vi "Get Last10 Data.vi"(8 "error in (no error)":errorcluster, 11 "Ref In":T1 {"TS Parameter"."FCA" format="%01d"; "TS Parameter"."Target" min=1 max=100000; "TS Parameter"."PokaYoke" min=0 max=1}) -> (0 "error out":errorcluster, 3 "Ref Out":T1 {"TS Parameter"."FCA" format="%01d"; "TS Parameter"."Target" min=1 max=100000; "TS Parameter"."PokaYoke" min=0 max=1}, 4 "BCODE SLNO":i32, 6 "Table Control":string[][](array[string]))   [LabVIEW 2020]
uses:
  Controls/TD SQL.ctl
  <vilib>/addons/database/Connection.llb/Conn ObjectReference.ctl
  Controls/WIP_State.ctl
  Controls/TS_Parameter.ctl
  <vilib>/addons/database/NI_Database_API.lvlib
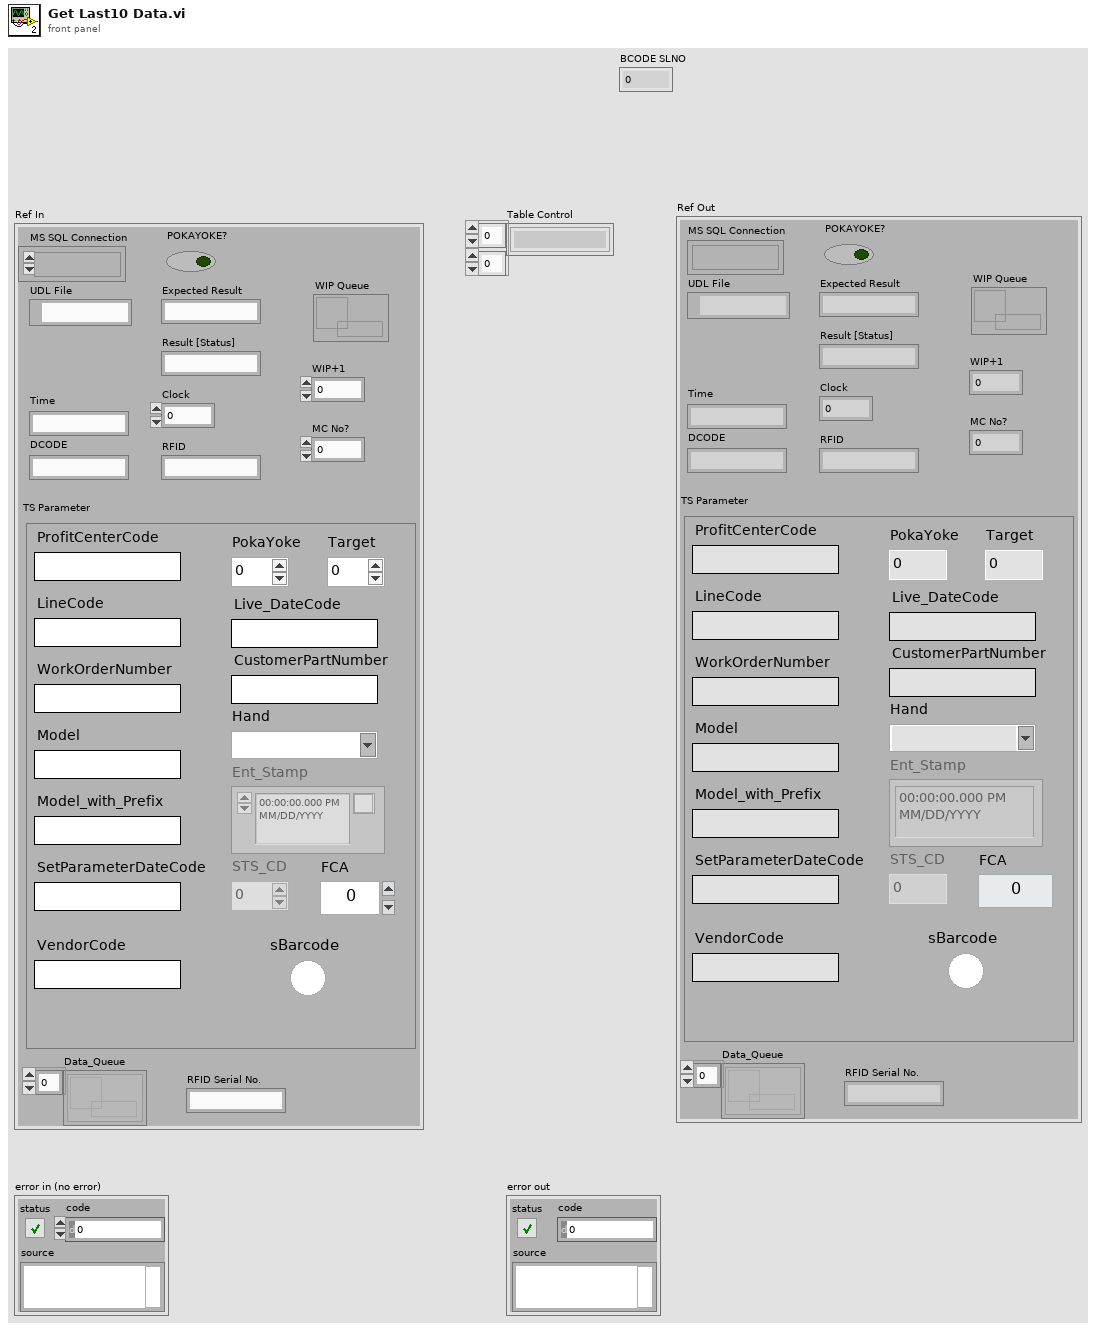
[diagram p1: front panel]
types:
  T1 = typedef "TD SQL.ctl" = cluster{"MS SQL Connection":T2, "UDL File":path, "Time":string, "DCODE":string, "WIP+1":i64, "MC No?":i32, "POKAYOKE?":bool, "Expected Result":string, "Result [Status]":string, "Clock":dbl, "RFID":string, "WIP Queue":refnum<queue>, "TS Parameter":T3, "Data_Queue":refnum<queue>[], "RFID Serial No.":string}
  T2 = typedef "NI_Database_API.lvlib/Conn ObjectReference.ctl" = refnum<k1>
  T3 = typedef "TS_Parameter.ctl" = cluster{"ProfitCenterCode":string, "LineCode":string, "WorkOrderNumber":string, "Model":string, "Model_with_Prefix":string, "VendorCode":string, "SetParameterDateCode":string, "PokaYoke":i32, "Target":i32, "Live_DateCode":string, "CustomerPartNumber":string, "Hand":string, "sBarcode":bool, "FCA":i32, "Ent_Stamp":timestamp, "STS_CD":dbl}
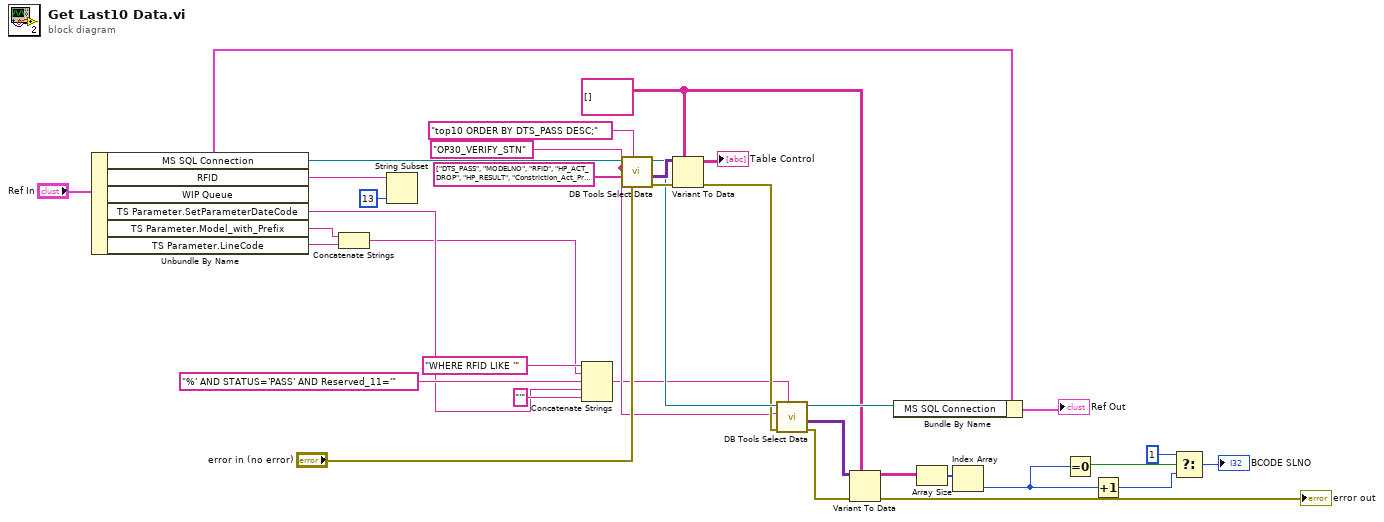
[diagram p0: block diagram]
diagram:
  w17 = string[][] [] ("Table Control")
  w22 = "OP30_VERIFY_STN" ("table")
  n1 = Unbundle By Name("Ref In") -> ("MS SQL Connection"=w28:T2, "RFID"=w13:string, "TS Parameter.SetParameterDateCode"=w5:string, "TS Parameter.Model_with_Prefix"=w4:string, "TS Parameter.LineCode"=w3:string)  [unwired: 1 out]
  n2 = Concatenate Strings(w4, w3) -> (w2:string)
  n3 = String Subset(string=w13, length (rest)=13 ("length (rest)")) -> ()  [unwired: 1 in, 1 out]
  n4 = Concatenate Strings("WHERE RFID LIKE '" ("string"), w2, "%' AND STATUS='PASS' AND Reserved_11='" ("condition"), w5, "'" ("string")) -> (w11:string)
  n5 = call <vilib>:"DB Tools Select Data.vi"("condition"="top10 ORDER BY DTS_PASS DESC;", "error in (no error)"="error in (no error)", "columns"=string[] ["DTS_PASS", "MODELNO", "RFID", "HP_ACT_DROP", "HP_RESULT", "Constriction_Act_Pr", "Constriction_Pr_Diff", "Constriction_Result", "CT", "Station_No"], "table"=w22, "connection reference"=w28) -> ("error out"=w33:errorcluster, "data"=w32:variant[][], "connection reference out"=w27:T2)  [unwired: 1 in]
  n6 = Variant To Data(error in=w33, type=w17, Variant=w32) -> (data=→"Table Control":string[][], error out=w26:errorcluster)
  n7 = call <vilib>:"DB Tools Select Data.vi"("condition"=w11, "error in (no error)"=w26, "table"=w22, "connection reference"=w27) -> ("error out"=w25:errorcluster, "data"=w24:variant[][], "connection reference out"=w20:T2)  [unwired: 2 in]
  n8 = Variant To Data(error in=w25, type=w17, Variant=w24) -> (data=w16:string[][], error out=→"error out":errorcluster)
  n9 = Bundle By Name(cluster="Ref In", "MS SQL Connection"=w20) -> (→"Ref Out":T1)
  n10 = Array Size(array=w16) -> (size(s)=w15:i32[])
  n11 = Index Array(array=w15) -> (element=w1:i32)  [unwired: 1 in]
  n12 = Equal To 0?(x=w1) -> (x = 0?=w10:bool)
  n13 = Increment(x=w1) -> (x+1=w9:i32)
  n14 = Select(t=1, s=w10, f=w9) -> (s? t:f=→"BCODE SLNO":i32)
